vi "generator współrzędnych GPS.vi"() -> ()   [LabVIEW 2015]
uses:
  <vilib>/Utility/file.llb/Read From Spreadsheet File (DBL).vi
  Zmienne/latitude.vi
  Zmienne/longitude.vi
  Zmienne globalne.lvlib
panel:
  in  "file path (dialog if empty)":path=path "C:/Users/User/Desktop/Pliki moduł map off-line 2/Testowe/quadron gps 2.txt"
  in  "stop":bool
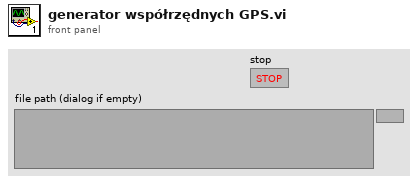
[diagram p1: front panel]
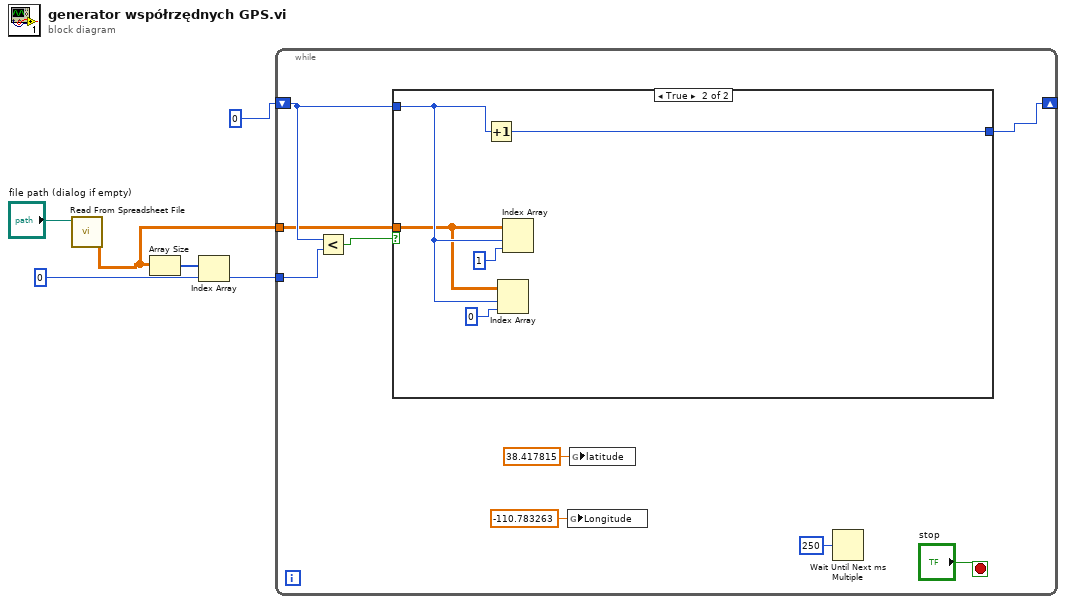
[diagram p0: block diagram]
diagram:
  n1 = call-poly <vilib>:"Read From Spreadsheet File.vi"("file path (dialog if empty)"="file path (dialog if empty)") -> ("all rows"=w1:dbl[][])  [unwired: 6 in, 4 out]
  n2 = Array Size(array=w1) -> (size(s)=w5:i32[])
  n3 = Index Array(array=w5, index=0) -> (element=w2:i32)
  n4 = while {
    shift-right: [w9] -> _
    shift-left: 0 ("index") -> [w11]
    tunnel: w2 -> [w13]
    tunnel: w1 -> [w10]
    stop <- "stop" stop-if-true
    n5 = Less?(x=w11, y=w13) -> (x < y?=w12:bool)
    n6 = case shown="True" w12 {
      tunnel: w11 -> [w16 w19]
      tunnel: w10 -> [_ w18]
      tunnel: [w16 w17] -> w9
      frame False {
      }
      frame True {
        n7 = Increment(x=w19) -> (x+1=w17:i32)
        n8 = Index Array(array=w18, index (row)=w19, index (col)=0) -> ()  [unwired: 1 out]
        n9 = Index Array(array=w18, index (row)=w19, index (col)=1 ("disabled index (col)")) -> ()  [unwired: 1 out]
      }
    }
    n10 = global write "longitude.vi" "Longitude"(-110.783263 ("Longitude")) -> ()
    n11 = global write "latitude.vi" "latitude"(38.417815 ("latitude")) -> ()
    n12 = Wait Until Next ms Multiple(millisecond multiple=u32 250) -> ()  [unwired: 1 out]
  }
